vi "MenuBuild.vi"(4 "Button\n(Mouse Down?)":u16, 5 "Clipboard":refnum<vi>, 6 "withinSelection?":bool=TRUE, 7 "row type":T1, 8 "error in (no error)":errorcluster, 9 "Table CtlRef In":refnum<vi>, 10 "MenuRef In":refnum<k9>, 11 "GroupCol in":refnum<class "GroupCol.lvclass">) -> (0 "error out":errorcluster, 1 "Table CtlRef Out":refnum<vi>, 2 "MenuRef Out":refnum<k9>, 3 "GroupCol out":refnum<class "GroupCol.lvclass">)   [LabVIEW 2013, in "GroupCol.lvclass"]
doc: "Build shortcut (right-click) menu items for Group column. This VI is read-only w.r.t column data."
uses:
  GroupCol.lvclass
  TypeDefs/RowType.ctl
  DigitalCol/DigitalCol.lvclass
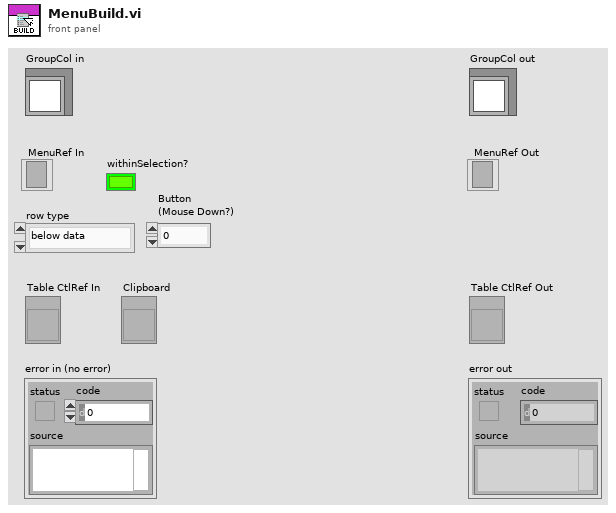
[diagram p1: front panel]
types:
  T1 = typedef "RowType.ctl" = enum16{"below data", "within data", "column header", "first row"}
  T2 = typedef "LVRowAndColumnTypeDef.ctl" = cluster{"Row":i32, "Column":i32}
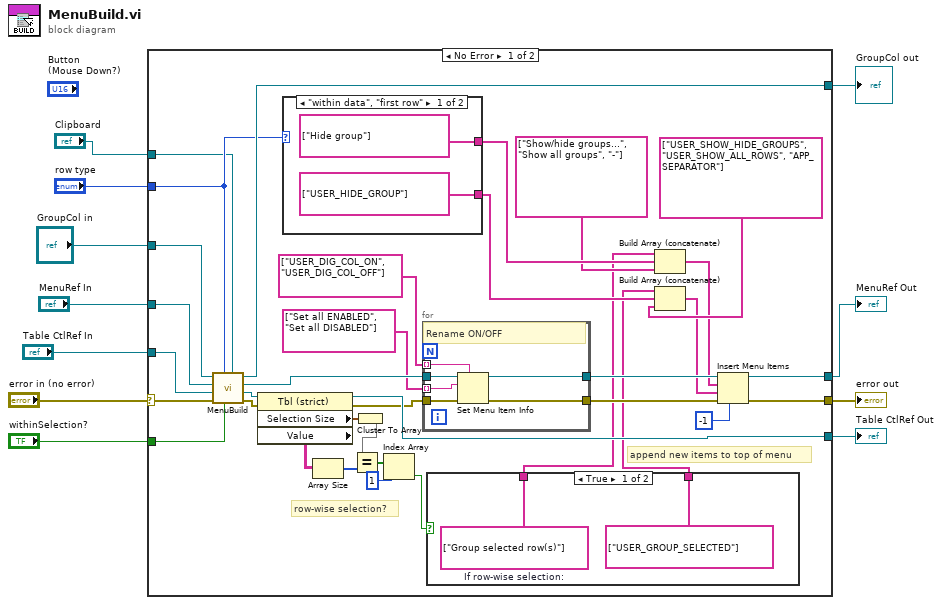
[diagram p0: block diagram]
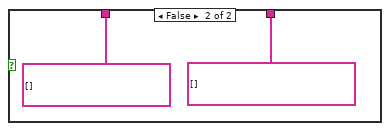
[diagram p2: hidden frame]
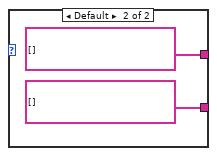
[diagram p3: hidden frame]
diagram:
  n1 = case shown="No Error" "error in (no error)" {
    selector: "error in (no error)" -> [w41 w61]
    tunnel: [w34 w61] -> w11
    tunnel: [w23 w62] -> w10
    tunnel: [w36 w63] -> w9
    tunnel: [w46 w64] -> w8
    tunnel: "row type" -> [w32 _]
    tunnel: "Table CtlRef In" -> [w45 w62]
    tunnel: "MenuRef In" -> [w44 w63]
    tunnel: "GroupCol in" -> [w43 w64]
    tunnel: "withinSelection?" -> [w42 _]
    tunnel: "Clipboard" -> [w25 _]
    frame No Error {
      # "row-wise selection?"
      # "append new items to top of menu"
      n2 = call-parent "MenuBuild.vi"("Clipboard"=w25, "withinSelection?"=w42, "row type"=w32, "error in (no error)"=w41, "Table CtlRef In"=w45, "MenuRef In"=w44, "DigitalCol in"=w43) -> ("error out"=w21:errorcluster, "Table CtlRef Out"=w24:refnum<vi>, "MenuRef Out"=w40:refnum<k9>, "DigitalCol out"=w46:refnum<class "GroupCol.lvclass">)  [unwired: 1 in]
      n3 = property class="Tbl (strict)"(reference=w24, error in=w21) -> (reference out=w23:refnum<vi>, error out=w22:errorcluster, "Selection Size"=w20:T2, "Value"=w19:string[][])
      n4 = case shown="\"within data\", \"first row\"" w32 {
        tunnel: [string[] ["Hide group"] string[] []] -> w27
        tunnel: [string[] ["USER_HIDE_GROUP"] string[] []] -> w31
        frame "within data", "first row" {
        }
        frame Default {
        }
      }
      n5 = Array Size(array=w19) -> (size(s)=w18:i32[])
      n6 = Cluster To Array(cluster=w20) -> (array=w17:i32[])
      n7 = Equal?(x=w17, y=w18) -> (x = y?=w16:bool[])
      n8 = Index Array(array=w16, index=1) -> (element=w12:bool)
      n9 = for {
        tunnel: w22 -> [w60]
        tunnel: [w59] -> w35
        tunnel: w40 -> [w58]
        tunnel: [w57] -> w37
        tunnel: string[] ["USER_DIG_COL_ON", "USER_DIG_COL_OFF"] -> [w56] mode=indexing
        tunnel: string[] ["Set all ENABLED", "Set all DISABLED"] -> [w55] mode=indexing
        # "Rename ON/OFF"
        n10 = Set Menu Item Info(7:w56, 8:w60, 10:w55, 11:w58) -> (0:w59:errorcluster, 3:w57:refnum<k9>)  [unwired: 3 in]
      }
      n11 = case shown="True" w12 {
        tunnel: [w48 string[] [] ("If row-wise selection:")] -> w13
        tunnel: [string[] ["USER_GROUP_SELECTED"] ("If in data bounds:") string[] [] ("If in data bounds:")] -> w14
        frame True {
          w48 = string[] ["Group selected row(s)"]  # If row-wise selection:
        }
        frame False {
        }
      }
      n12 = Build Array (concatenate)(w13, w27, string[] ["Show/hide groups...", "Show all groups", "-"]) -> (w28:string[])
      n13 = Build Array (concatenate)(w14, w31, string[] ["USER_SHOW_HIDE_GROUPS", "USER_SHOW_ALL_ROWS", "APP_SEPARATOR"]) -> (w29:string[])
      n14 = Insert Menu Items(4:-1, 6:w35, 7:w29, 8:w28, 9:w37) -> (0:w34:errorcluster, 3:w36:refnum<k9>)  [unwired: 1 in, 1 out]
    }
    frame Error {
    }
  }
  "error out" <- w11
  "GroupCol out" <- w8
  "MenuRef Out" <- w9
  "Table CtlRef Out" <- w10
